vi "GlobalSender.vi"() -> ()   [LabVIEW 2015]
panel:
  in  "String":string
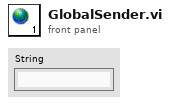
[diagram p1: front panel]
diagram:
